vi "_VIServerRefType.vi"(4 "Data":variant) -> (1 "Enum":T1(ring)=enum."VI")   [LabVIEW 2017, in "TagDB.lvlib"]
doc: "Gets the Refnum Type Enumeration of the input."
uses:
  TagDB.lvlib
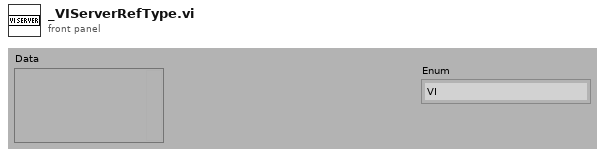
[diagram p1: front panel]
types:
  T1 = enum16{"Not a VI Server Refnum", "Control", "VI", "Application", "Splitter", "Pane"}
  T2 = enum8{"Generic", "Datalog File Refnum", "Byte Stream File Refnum", "Device Refnum", "Occurence Refnum", "TCP Connection Refnum", "VISA Refnum (Obsolete)", "Automation Renum", "VI Server Refnum", "Menu Refnum", "IVI Refnum (Obsolete)", "IMAQ Session", "0x0C", "Datasocket Refnum", "VISA Resource", "IVI Logical Name", "UDP Connection Refnum", "Notifier Refnum", "Queue Refnum", "IrDA Refnum", "Hardware Plugin Refnum", "Hardware Plugin Tag Refnum", "DAQmx Refnum", "Event Registration Refnum", ".NET Refnum", "User Event Refnum", "0x1A", "Event Callback", "0x1C", "0x1D", "Only Used Internal to LabVIEW", "Bluetooth", "Data Value References", "RT FIFO", "TDM Streaming"}
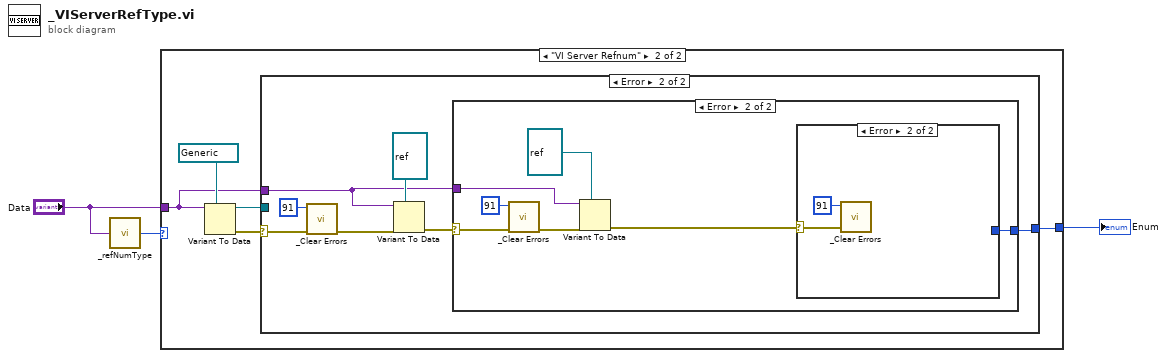
[diagram p0: block diagram]
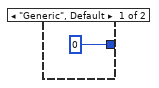
[diagram p2: hidden frame]
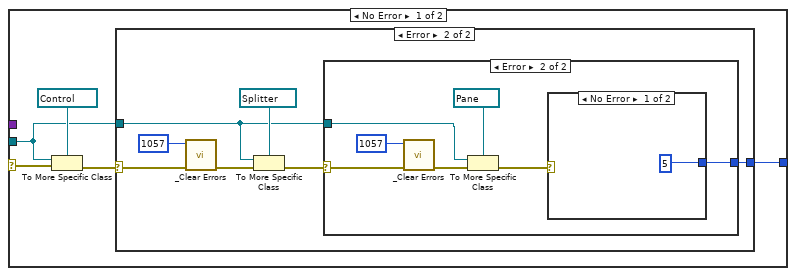
[diagram p3: hidden frame]
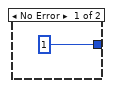
[diagram p4: hidden frame]
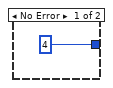
[diagram p5: hidden frame]
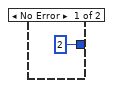
[diagram p7: hidden frame]
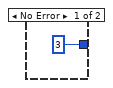
[diagram p8: hidden frame]
diagram:
  n1 = call "_refNumType.vi"("Data"="Data") -> ("Refnum Subtype Enum"=w2:T2)  [unwired: 4 in]
  n2 = case shown="\"VI Server Refnum\"" w2 {
    tunnel: "Data" -> [_ w6]
    tunnel: [0 w5] -> w1
    frame "Generic", Default {
    }
    frame "VI Server Refnum" {
      n3 = Variant To Data(type=refnum<vi> refnum ("Data"), Variant=w6) -> (data=w8:refnum<vi>, error out=w9:errorcluster)  [unwired: 1 in]
      n4 = case shown="Error" w9 {
        selector: w9 -> [w10 w37]
        tunnel: w8 -> [w11 _]
        tunnel: w6 -> [_ w32]
        tunnel: [w14 w33] -> w5
        frame No Error {
          n5 = To More Specific Class(target class=refnum<vi> refnum ("Data"), reference=w11, error in=w10) -> (error out=w12:errorcluster)  [unwired: 1 out]
          n6 = case shown="Error" w12 {
            selector: w12 -> [_ w21]
            tunnel: [1 w17] -> w14
            tunnel: w11 -> [_ w16]
            frame No Error {
            }
            frame Error {
              n7 = call "_Clear Errors.vi"("error in (no error)"=w21, "specific error code to clear (0: all)"=1057) -> ("error out"=w20:errorcluster)  [unwired: 4 in, 1 out]
              n8 = To More Specific Class(target class=refnum<vi> refnum ("Data"), reference=w16, error in=w20) -> (error out=w18:errorcluster)  [unwired: 1 out]
              n9 = case shown="Error" w18 {
                selector: w18 -> [_ w29]
                tunnel: [4 w25] -> w17
                tunnel: w16 -> [_ w26]
                frame No Error {
                }
                frame Error {
                  n10 = call "_Clear Errors.vi"("error in (no error)"=w29, "specific error code to clear (0: all)"=1057) -> ("error out"=w27:errorcluster)  [unwired: 4 in, 1 out]
                  n11 = To More Specific Class(target class=refnum<vi> refnum ("Data"), reference=w26, error in=w27) -> (error out=w24:errorcluster)  [unwired: 1 out]
                  n12 = case shown="No Error" w24 {
                    tunnel: [5 _] -> w25
                    frame No Error {
                    }
                    frame Error {
                    }
                  }
                }
              }
            }
          }
        }
        frame Error {
          n13 = call "_Clear Errors.vi"("error in (no error)"=w37, "specific error code to clear (0: all)"=91) -> ("error out"=w36:errorcluster)  [unwired: 4 in, 1 out]
          n14 = Variant To Data(error in=w36, type=refnum<vi> refnum ("This VI"), Variant=w32) -> (error out=w34:errorcluster)  [unwired: 1 out]
          n15 = case shown="Error" w34 {
            selector: w34 -> [_ w44]
            tunnel: [2 w40] -> w33
            tunnel: w32 -> [_ w43]
            frame No Error {
            }
            frame Error {
              n16 = call "_Clear Errors.vi"("error in (no error)"=w44, "specific error code to clear (0: all)"=91) -> ("error out"=w45:errorcluster)  [unwired: 4 in, 1 out]
              n17 = Variant To Data(error in=w45, type=refnum<vi> refnum ("application reference"), Variant=w43) -> (error out=w41:errorcluster)  [unwired: 1 out]
              n18 = case shown="Error" w41 {
                selector: w41 -> [_ w48]
                tunnel: [3 _] -> w40
                frame No Error {
                }
                frame Error {
                  n19 = call "_Clear Errors.vi"("error in (no error)"=w48, "specific error code to clear (0: all)"=91) -> ()  [unwired: 4 in, 2 out]
                }
              }
            }
          }
        }
      }
    }
  }
  "Enum" <- w1
